vi "get channel index by id.vi"(8 "error in (no error)":errorcluster, 10 "id":string, 11 "configuration file cluster in":T1) -> (0 "error out":errorcluster, 1 "found?":bool, 2 "index":i32, 3 "configuration file cluster out":T1)   [LabVIEW 2017, in "DSF Configuration API v1.0.0.lvlib"]
uses:
  DSF Configuration API v1.0.0.lvlib
  Controls/dsf configuration file/1.0.0/DSF Channel.ctl
  File API/DSFConfig.lvlib
  Controls/dsf configuration file/1.0.0/DSF Transfer.ctl
  Controls/dsf configuration file/1.0.0/dsf timing.ctl
  Controls/dsf configuration file/1.0.0/DSF Group.ctl
  Controls/dsf configuration file/1.0.0/DSF Plugin.ctl
  Controls/dsf configuration file/1.0.0/Version Info.ctl
  Controls/dsf configuration file/1.0.0/DSF Settings.ctl
  Controls/dsf configuration file/1.0.0/DSF Config.ctl
  Controls/dsf configuration file/1.0.0/DSF Channel Info.ctl
  Controls/dsf configuration file/1.0.0/DSF Settings Info.ctl
  Controls/dsf configuration file/1.0.0/DSF Transfer Info.ctl
  File API/DSF Plugin Info.ctl
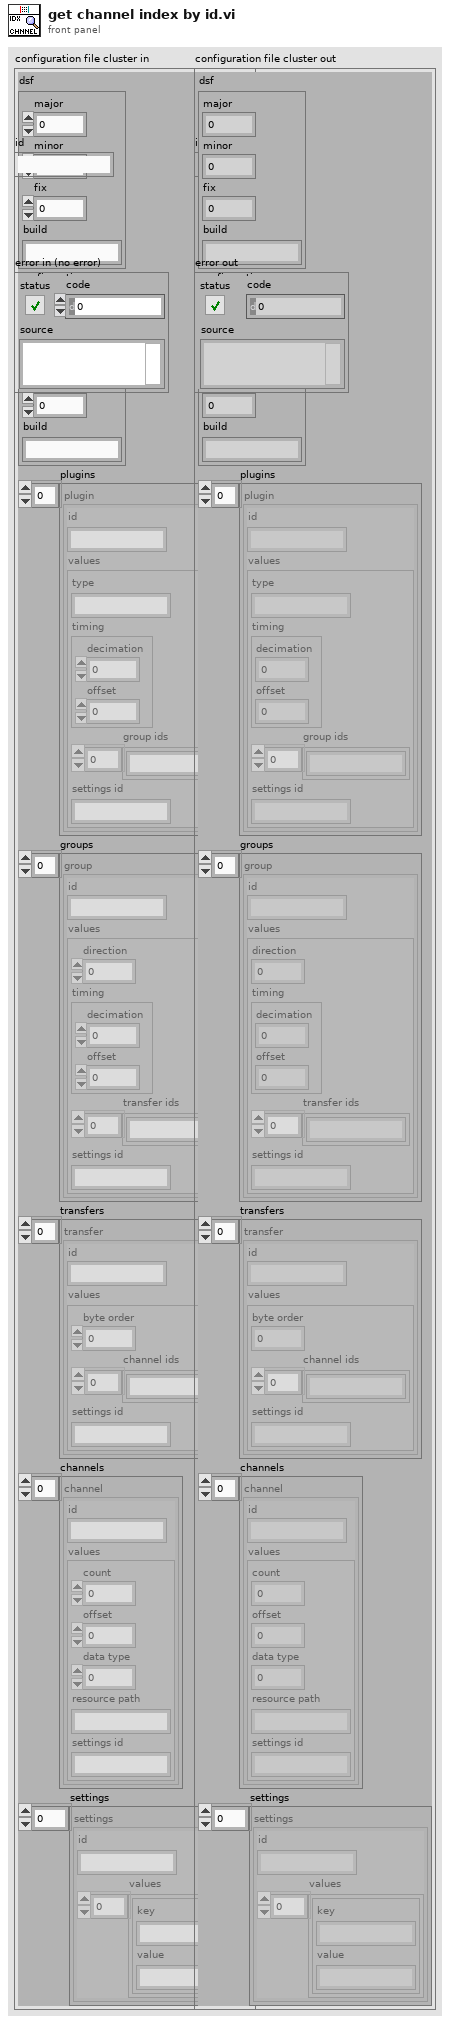
[diagram p1: front panel]
types:
  T1 = typedef "DSFConfig.lvlib/DSF Config.ctl" = cluster{"dsf":T2, "configuration":T2, "plugins":T3[], "groups":T6[], "transfers":T7[], "channels":T9[], "settings":T11[]}
  T2 = typedef "DSFConfig.lvlib/Version Info.ctl" = cluster{"major":u32, "minor":u32, "fix":u32, "build":string}
  T3 = typedef "DSFConfig.lvlib/DSF Plugin.ctl" = cluster{"id":string, "values":T4}
  T4 = typedef "DSFConfig.lvlib/DSF Plugin Info.ctl" = cluster{"type":string, "timing":T5, "group ids":string[], "settings id":string}
  T5 = typedef "DSFConfig.lvlib/dsf timing.ctl" = cluster{"decimation":i32, "offset":i32}
  T6 = typedef "DSFConfig.lvlib/DSF Group.ctl" = cluster{"id":string, "values":cluster{"direction":i32, "timing":T5, "transfer ids":string[], "settings id":string}}
  T7 = typedef "DSFConfig.lvlib/DSF Transfer.ctl" = cluster{"id":string, "values":T8}
  T8 = typedef "DSFConfig.lvlib/DSF Transfer Info.ctl" = cluster{"byte order":i32, "channel ids":string[], "settings id":string}
  T9 = typedef "DSFConfig.lvlib/DSF Channel.ctl" = cluster{"id":string, "values":T10}
  T10 = typedef "DSFConfig.lvlib/DSF Channel Info.ctl" = cluster{"count":i32, "offset":i32, "data type":i32, "resource path":string, "settings id":string}
  T11 = typedef "DSFConfig.lvlib/DSF Settings.ctl" = cluster{"id":string, "values":T12}
  T12 = typedef "DSFConfig.lvlib/DSF Settings Info.ctl" = cluster{"key":string, "value":string}[]
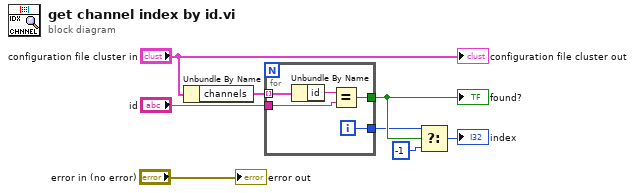
[diagram p0: block diagram]
diagram:
  n1 = Unbundle By Name("configuration file cluster in") -> ("channels"=w8:T9[])
  n2 = for {
    tunnel: w8 -> [w13] mode=indexing
    tunnel: "id" -> [w11]
    tunnel: [w10] -> w5
    tunnel: [w9] -> w3
    i -> [w9]
    n3 = Unbundle By Name(w13) -> ("id"=w12:string)
    n4 = Equal?(x=w12, y=w11) -> (x = y?=w10:bool)
  }
  "found?" <- w5
  n5 = Select(t=w3, s=w5, f=-1) -> (s? t:f=→"index":i32)
  "configuration file cluster out" <- "configuration file cluster in"
  "error out" <- "error in (no error)"
